vi "Generate Intensities.vi"(9 "eta*cosalpha":dbl=-0.0303, 10 "Lorentzian Width":dbl=0.05, 11 "R":dbl) -> (3 "Intensity":dbl)   [LabVIEW 2019]
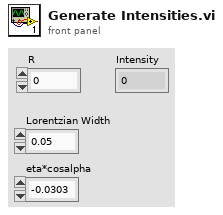
[diagram p1: front panel]
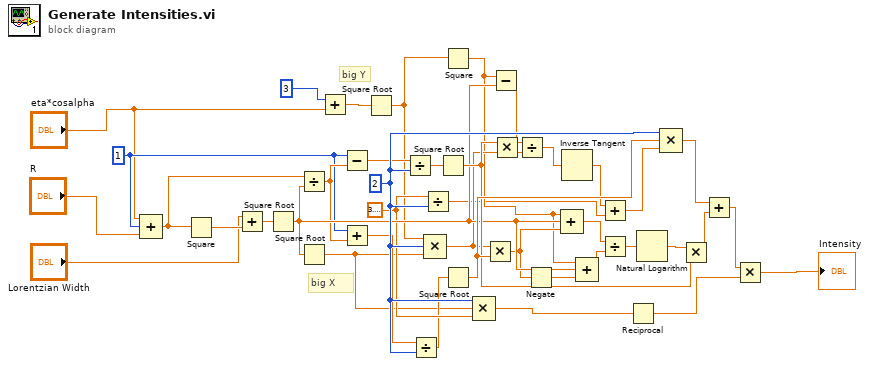
[diagram p0: block diagram]
diagram:
  w19 = 3.141592653589793
  w35 = 2
  w16 = 1
  # "big X"
  # "big Y"
  n1 = Compound Arithmetic op=ADD("eta*cosalpha", w16, "R") -> (w10:dbl)
  n2 = Square(x=w10) -> (x^2=w8:dbl)
  n3 = Add(x="Lorentzian Width", y=w8) -> (x+y=w9:dbl)
  n4 = Square Root(x=w9) -> (sqrt(x)=w29:dbl)
  n5 = Divide(x=w10, y=w29) -> (x/y=w17:dbl)
  n6 = Square Root(x=w29) -> (sqrt(x)=w4:dbl)
  n7 = Add(x=3, y="eta*cosalpha") -> (x+y=w1:dbl)
  n8 = Subtract(x=w16, y=w17) -> (x-y=w12:dbl)
  n9 = Add(x=w16, y=w17) -> (x+y=w11:dbl)
  n10 = Square Root(x=w1) -> (sqrt(x)=w6:dbl)
  n11 = Divide(x=w12, y=w35) -> (x/y=w15:dbl)
  n12 = Divide(x=w11, y=w35) -> (x/y=w14:dbl)
  n13 = Divide(x=w19, y=w35) -> (x/y=w24:dbl)
  n14 = Compound Arithmetic op=MULTIPLY(w6, w35, w4) -> (w27:dbl)
  n15 = Square Root(x=w15) -> (sqrt(x)=w34:dbl)
  n16 = Square(x=w6) -> (x^2=w26:dbl)
  n17 = Square Root(x=w14) -> (sqrt(x)=w36:dbl)
  n18 = Compound Arithmetic op=MULTIPLY(w35, w4, w19) -> (w18:dbl)
  n19 = Multiply(x=w27, y=w36) -> (x*y=w28:dbl)
  n20 = Subtract(x=w26, y=w29) -> (x-y=w20:dbl)
  n21 = Multiply(x=w34, y=w27) -> (x*y=w21:dbl)
  n22 = Divide(x=w20, y=w21) -> (x/y=w22:dbl)
  n23 = Negate(x=w28) -> (-x=w25:dbl)
  n24 = Compound Arithmetic op=ADD(w26, w29, w28) -> (w30:dbl)
  n25 = Inverse Tangent(1:w22) -> (0:w23:dbl)
  n26 = Compound Arithmetic op=ADD(w26, w29, w25) -> (w31:dbl)
  n27 = Add(x=w23, y=w24) -> (x+y=w37:dbl)
  n28 = Divide(x=w30, y=w31) -> (x/y=w32:dbl)
  n29 = Reciprocal(x=w18) -> (1/x=w41:dbl)
  n30 = Natural Logarithm(1:w32) -> (0:w33:dbl)
  n31 = Compound Arithmetic op=MULTIPLY(w35, w36, w37) -> (w38:dbl)
  n32 = Multiply(x=w33, y=w34) -> (x*y=w39:dbl)
  n33 = Add(x=w38, y=w39) -> (x+y=w40:dbl)
  n34 = Multiply(x=w40, y=w41) -> (x*y=→"Intensity":dbl)
